vi "RedVi.vi"() -> ()   [LabVIEW 2017]
panel:
  in  "Ctl Refnum":refnum<vi>
  out "String":string
  in  "Boolean":bool
  in  "Path":path
  in  "Numeric":dbl
  in  "Run Test":bool
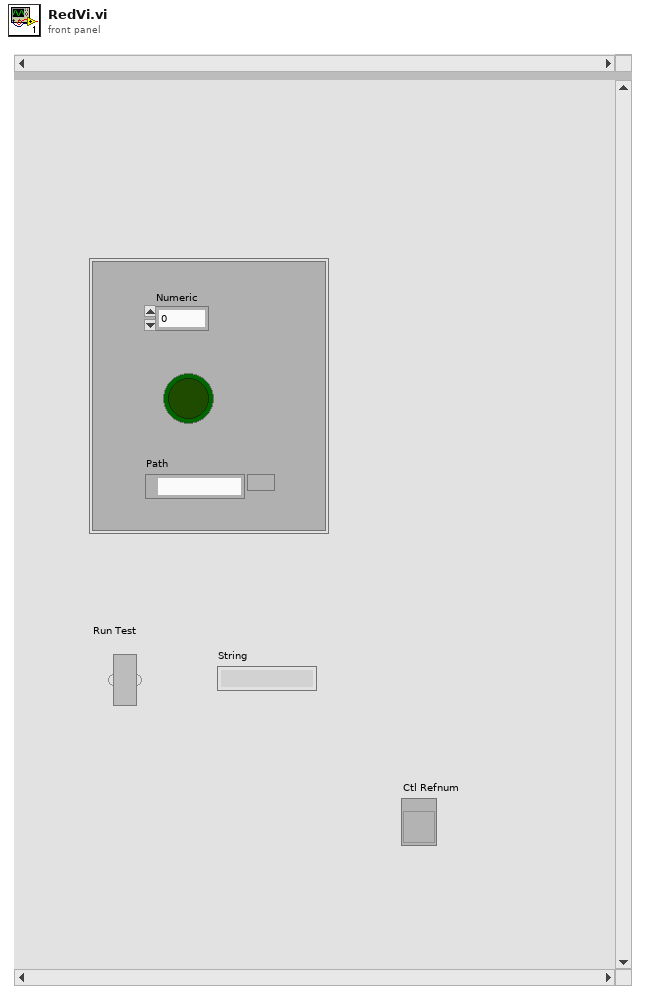
[diagram p1: front panel]
types:
  T1 = enum8{"Enabled", "Disabled", "Disabled and Grayed Out"}
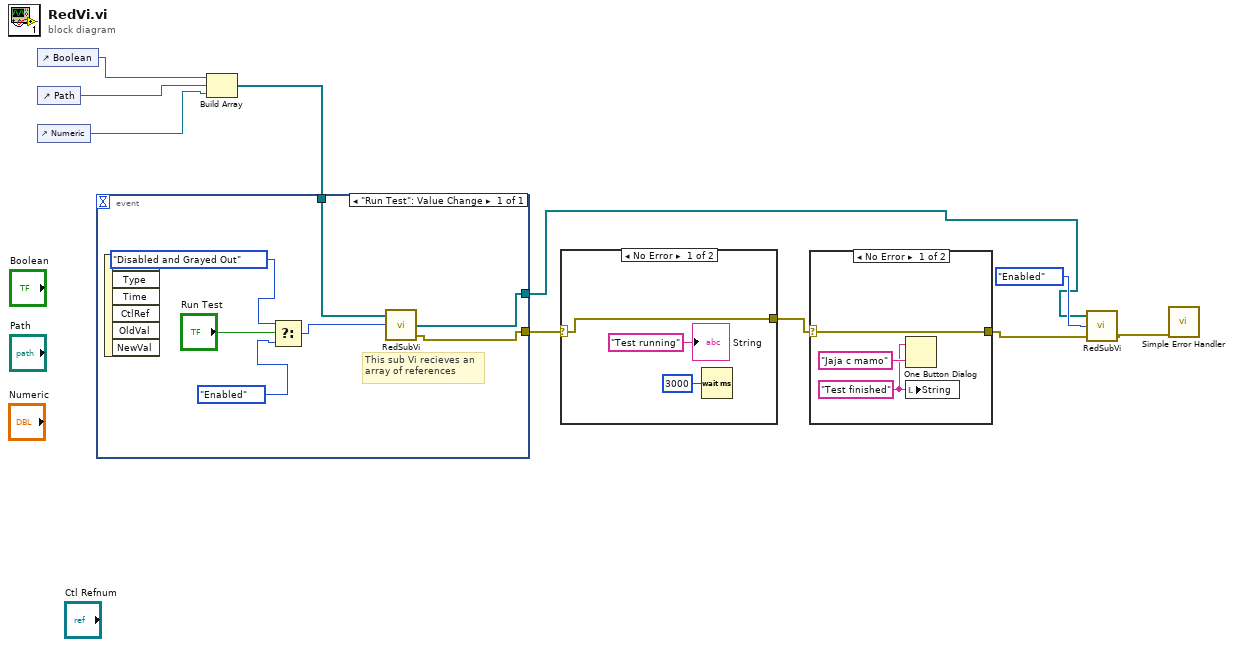
[diagram p0: block diagram]
diagram:
  n1 = control-ref of="Boolean"() -> (w10:refnum<vi>)
  n2 = control-ref of="Path"() -> (w9:refnum<vi>)
  n3 = control-ref of="Numeric"() -> (w8:refnum<vi>)
  n4 = Build Array(w10, w9, w8) -> (w5:refnum<vi>[])
  n5 = event shown="[0] \"Run Test\": Value Change" {
    selector: _ -> [_]
    dyn-events: _ -> [_]
    timeout: _ -> [_]
    tunnel: w5 -> [w14]
    tunnel: [w12] -> w7
    tunnel: [w11] -> w1
    event "Run Test": Value Change {
      # "This sub Vi recieves an\narray of references"
      n6 = event-data() -> ()  [unwired: 1 in, 6 out]
      n7 = Select(t=T1."Disabled and Grayed Out" ("Disabled"), s="Run Test", f=T1."Enabled" ("Disabled")) -> (s? t:f=w13:T1)
      n8 = call "RedSubVi.vi"("Disabled"=w13, "Array"=w14) -> ("error out"=w12:errorcluster, "Output reference"=w11:refnum<vi>[])  [unwired: 2 in]
    }
  }
  n9 = case shown="No Error" w7 {
    selector: w7 -> [w18 w21]
    tunnel: [w18 w21] -> w6
    frame No Error {
      n10 = Wait (ms)(milliseconds to wait=u32 3000) -> ()  [unwired: 1 out]
      "String" <- "Test running" ("String")
    }
    frame Error {
    }
  }
  n11 = case shown="No Error" w6 {
    selector: w6 -> [w23 w25]
    tunnel: [w23 w25] -> w3
    frame No Error {
      w22 = "Test finished" ("message")
      n12 = One Button Dialog(message=w22, button name ("OK")="Jaja c mamo") -> ()  [unwired: 1 out]
      n13 = local write "String"(w22) -> ()
    }
    frame Error {
    }
  }
  n14 = call "RedSubVi.vi"("error in (no error)"=w3, "Disabled"=T1."Enabled", "Array"=w1) -> ("error out"=w4:errorcluster)  [unwired: 1 in, 1 out]
  n15 = call <vilib>:"Simple Error Handler.vi"("error in (no error)"=w4) -> ()  [unwired: 4 in, 5 out]
